vi "Retrieve_Signal_Level.vi"() -> ()   [LabVIEW 2020]
panel:
  in  "reference":refnum<vi>
  out "error out":errorcluster
  out "Oscillator Signal Level":dbl
  in  "OK Button":bool
  in  "error in (no error)":errorcluster
  # "Adjust OSC LEVEL (V) to desired level"
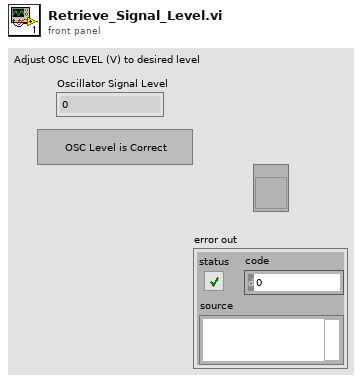
[diagram p1: front panel]
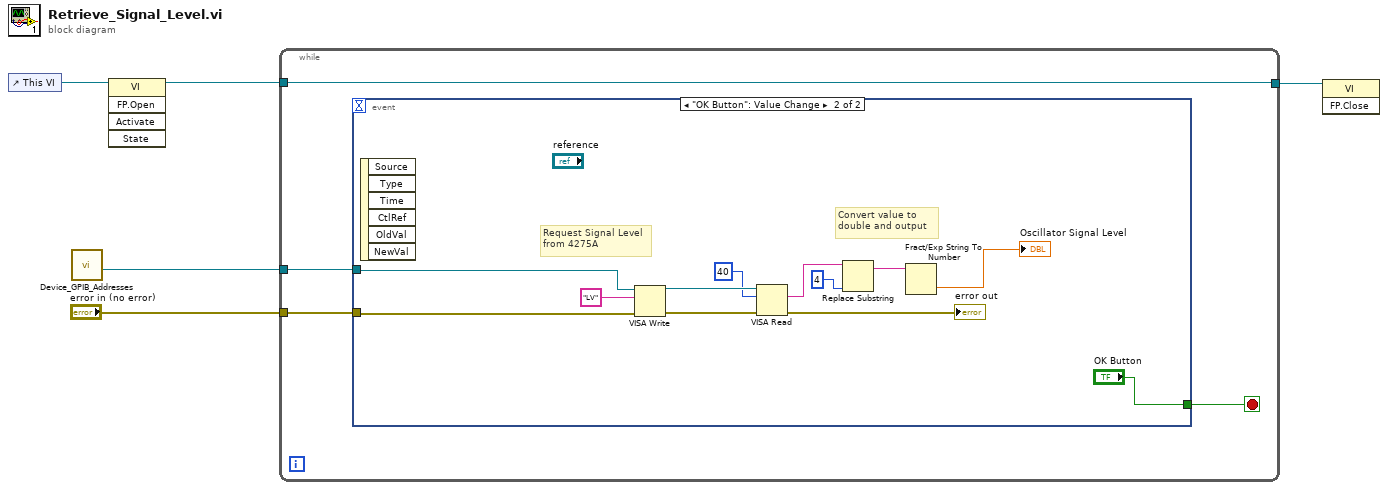
[diagram p0: block diagram]
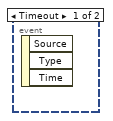
[diagram p2: hidden frame]
diagram:
  n1 = control-ref of="This VI"() -> (w3:refnum<vi>)
  n2 = call "Device_GPIB_Addresses.vi"() -> ("HP 4275A Address"=w4:refnum<visa-resource-name>)  [unwired: 9 in, 2 out]
  n3 = invoke on="Invoke Node" class="VI" method="FP.Open"(reference=w3) -> (reference out=w2:refnum<vi>)  [unwired: 4 in, 4 out]
  n4 = while {
    tunnel: "error in (no error)" -> [w9]
    tunnel: w4 -> [w8]
    tunnel: [w7] -> w1
    tunnel: w2 -> [w7]
    stop <- w6 stop-if-true
    n5 = event shown="[1] \"OK Button\": Value Change" {
      selector: _ -> [_ _]
      dyn-events: _ -> [_ _]
      timeout: _ -> [_ _]
      tunnel: w9 -> [_ w11]
      tunnel: w8 -> [_ w12]
      tunnel: [_ "OK Button"] -> w6
      event Timeout {
        n6 = event-data() -> ()  [unwired: 1 in, 3 out]
      }
      event "OK Button": Value Change {
        # "Convert value to\ndouble and output"
        # "Request Signal Level\nfrom 4275A"
        n7 = event-data() -> ()  [unwired: 1 in, 6 out]
        n8 = VISA Write(VISA resource name=w12, write buffer="LV", error in (no error)=w11) -> (VISA resource name out=w20:refnum<visa-resource-name>, error out=w19:errorcluster)  [unwired: 1 out]
        n9 = VISA Read(VISA resource name=w20, byte count=u32 40, error in (no error)=w19) -> (read buffer=w16:string, error out=→"error out":errorcluster)  [unwired: 2 out]
        n10 = Replace Substring(2:4 ("length (len. of substring)"), 5:w16) -> (1:w15:string)  [unwired: 2 in, 1 out]
        n11 = Fract/Exp String To Number(string=w15) -> (number=→"Oscillator Signal Level":dbl)  [unwired: 3 in, 1 out]
      }
    }
  }
  n12 = invoke on="Invoke Node" class="VI" method="FP.Close"(reference=w1) -> ()  [unwired: 2 in, 3 out]
